vi "RT Main.vi"() -> ()   [LabVIEW 2018]
uses:
  FPGA Bitfile Register Operations/Scalar IO Operations/TypeDefs/FXP Configuration.ctl
  <vilib>/fxp/LVFixedPointRepBitsTypeDef.ctl
  <vilib>/fxp/LVFixedPointRepRangeTypeDef.ctl
  FPGA Bitfile Register Operations/Scalar IO Operations/Read Methods/Read FXP.vi
  <vilib>/FPGAPlugInAG/Dynamic/niLvFpga_Close_Dynamic.vi
  <vilib>/rvi/interface/nirviCloseFPGA/nirviCloseFPGA.xnode
  FPGA Bitfile Register Operations/Scalar IO Operations/Scalar IO Operations.lvlib
panel:
  out "Average seconds per read":dbl
  out "Value":dbl
  out "error out":errorcluster
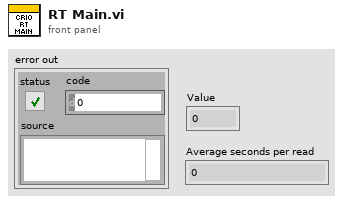
[diagram p1: front panel]
types:
  T1 = typedef "Scalar IO Operations.lvlib/FXP Configuration.ctl" = cluster{"FXP Representation":T2, "FXP Range":T3}
  T2 = typedef "LVFixedPointRepBitsTypeDef.ctl" = cluster{"Signed":bool, "Word Length":u32, "Integer Word Length":i32}
  T3 = typedef "LVFixedPointRepRangeTypeDef.ctl" = cluster{"Range Min":dbl, "Range Max":dbl, "Delta":dbl}
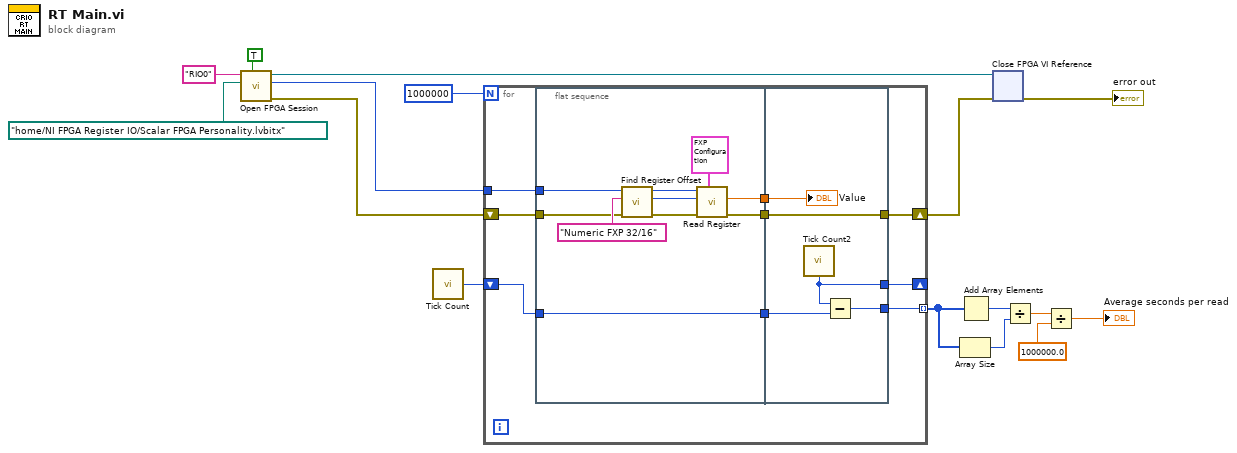
[diagram p0: block diagram]
diagram:
  n1 = call "Open FPGA Session.vi"("run when loaded (T)"=TRUE ("Run When Loaded (T)"), "bitfile path"=path "/home/NI FPGA Register IO/Scalar FPGA Personality.lvbitx" ("Bitfile path"), "device address"="RIO0" ("Device address")) -> ("error out"=w1:errorcluster, "session out"=w2:u64, "bitfile reference out"=w4:refnum<k20>)  [unwired: 6 in]
  n2 = call "Tick Count"() -> ("Tick Count(uSec)"=w11:u32)
  n3 = for {
    N: 1000000 -> [_]
    tunnel: w2 -> [w25]
    shift-right: [w23] -> w13
    shift-left: w1 -> [w24]
    shift-right: [w19] -> _
    shift-left: w11 -> [w21]
    tunnel: [w18] -> w10 mode=indexing
    n4 = flat-sequence {
      tunnel: w25 -> [w31]
      tunnel: w24 -> [w30]
      tunnel: [w35] -> w22
      tunnel: w21 -> [w34]
      tunnel: [w34] -> w20
      tunnel: [w33] -> w17
      tunnel: [w40] -> w23
      tunnel: w22 -> [w40]
      tunnel: w20 -> [w39]
      tunnel: [w38] -> w19
      tunnel: [w37] -> w18
      tunnel: w17 -> [w36]
      frame #0 {
        n5 = call "Find Register Offset.vi"("error in (no error)"=w30, "register name"="Numeric FXP 32/16" ("registerName"), "session in"=w31) -> ("error out"=w29:errorcluster, "resource offset"=w27:u32, "session out"=w28:u32)  [unwired: 6 in]
        n6 = call-poly "Read Register.vi"("FXP Configuration"=T1 {"FXP Representation"={"Signed"=TRUE, "Word Length"=32, "Integer Word Length"=0}, "FXP Range"={"Range Min"=0.0, "Range Max"=0.0, "Delta"=1.52588e-05}}, "error in"=w29, "register offset"=w27, "session in"=w28) -> ("error out"=w35:errorcluster, "DBL Value"=w33:dbl)  [unwired: 5 in, 1 out]
      }
      frame #1 {
        n7 = call "Tick Count2"() -> ("Tick Count(uSec)"=w38:u32)
        n8 = Subtract(x=w38, y=w39) -> (x-y=w37:u32)
        "Value" <- w36
      }
    }
  }
  n9 = Array Size(array=w10) -> (size(s)=w8:i32)
  n10 = Add Array Elements(numeric array=w10) -> (sum=w9:u32)
  n11 = xnode "Close FPGA VI Reference"("FPGA VI Reference In"=w4, "error in"=w13) -> ("error out"=→"error out":errorcluster)
  n12 = Divide(x=w9, y=w8) -> (x/y=w7:dbl)
  n13 = Divide(x=w7, y=1000000.0) -> (x/y=→"Average seconds per read":dbl)
